vi "Get Plugin Configurations.vi"(8 "error in (no error)":errorcluster, 11 "Framework Configuration in":refnum<class "Framework Configuration.lvclass">) -> (0 "error out":errorcluster, 2 "Plugin Configurations":refnum<class "Plugin Configuration.lvclass">[](array[class]), 3 "Framework Configuration out":refnum<class "Framework Configuration.lvclass">)   [LabVIEW 2017, in "DSF Core.lvlib" / "Framework Configuration.lvclass"]
uses:
  Framework Configuration.lvclass
  Plugin/Plugin Configuration.lvclass
  Framework Configuration.lvclass/Framework Configuration.ctl
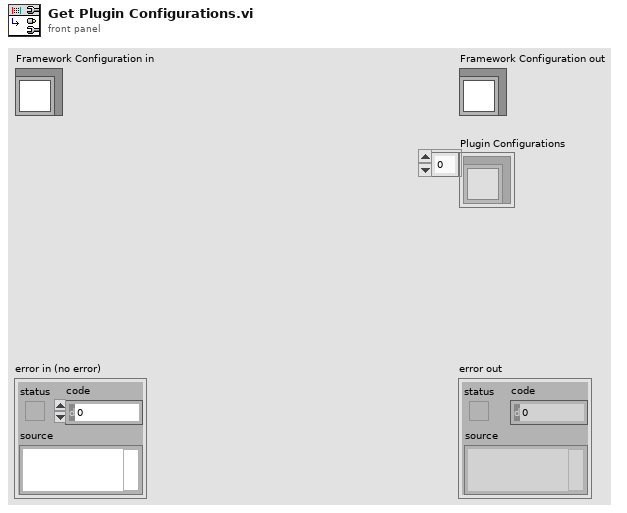
[diagram p1: front panel]
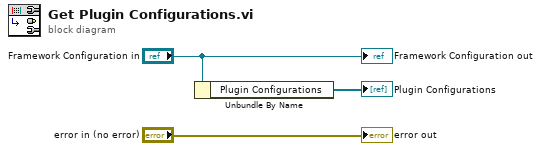
[diagram p0: block diagram]
diagram:
  n1 = Unbundle By Name("Framework Configuration in") -> ("Plugin Configurations"=→"Plugin Configurations":refnum<class "Plugin Configuration.lvclass">[])
  "error out" <- "error in (no error)"
  "Framework Configuration out" <- "Framework Configuration in"
